vi "LV RT Doc - Instantiate with Path.vi"(5 "LV Doc Path":path, 11 "error in (no error)":errorcluster) -> (4 "Document out":refnum<class "Document.lvclass">, 15 "error out":errorcluster)   [LabVIEW 2016, in "LV RT.lvclass"]
uses:
  LV RT.lvclass
  Document.lvclass
  C:/Users/namratha.balakrishna/Desktop/source code/MDI/D/MDI Project/source code/Document/Document.lvclass
  Document.lvclass/Document.ctl
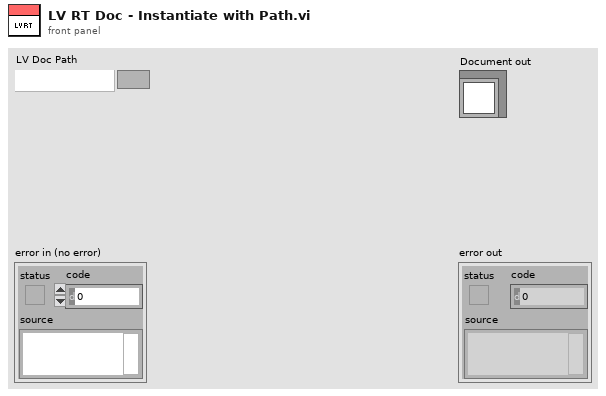
[diagram p1: front panel]
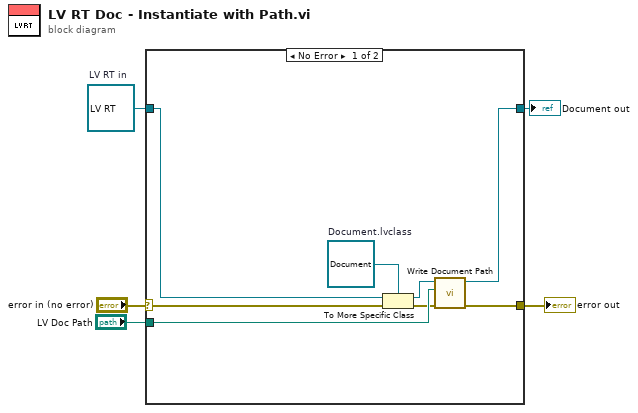
[diagram p0: block diagram]
diagram:
  w3 = refnum<class "LV RT.lvclass"> refnum  # LV RT in
  n1 = case shown="No Error" "error in (no error)" {
    selector: "error in (no error)" -> [w13 w15]
    tunnel: [w11 w15] -> w4
    tunnel: [w10 w14] -> w1
    tunnel: w3 -> [w12 w14]
    tunnel: "LV Doc Path" -> [w9 _]
    frame No Error {
      w8 = refnum<class "Document.lvclass"> refnum  # Document.lvclass
      n2 = To More Specific Class(target class=w8, reference=w12, error in=w13) -> (specific class reference=w7:refnum<class "Document.lvclass">, error out=w6:errorcluster)
      n3 = call "Write Document Path.vi"("error in (no error)"=w6, "Document Path"=w9, "Document in"=w7) -> ("error out"=w11:errorcluster, "Document out"=w10:refnum<class "Document.lvclass">)  [unwired: 7 in]
    }
    frame Error {
    }
  }
  "error out" <- w4
  "Document out" <- w1
